vi "PathFollowingFinal.vi"(0 "GPS_Lat":dbl format="%#_13g", 5 "GPS_Long":dbl format="%#_13g", 7 "Path":dbl[][](array[numeric]), 9 "Heading angle":dbl, 11 "Save heading":bool=TRUE) -> (4 "Path rest":dbl[][](array[numeric]), 6 "Delta Heading Angle":dbl, 8 "Goal reached":bool, 10 "Beta":dbl format="%#_13g")   [LabVIEW 2016]
uses:
  <vilib>/express/express arith-compare/Formula/XNode/ExpressFormulaBlockNode.xnode
panel:
  out "Angle":dbl
  out "Distance":dbl format="%#.14g"
  out "Next Point":dbl[](array[numeric])
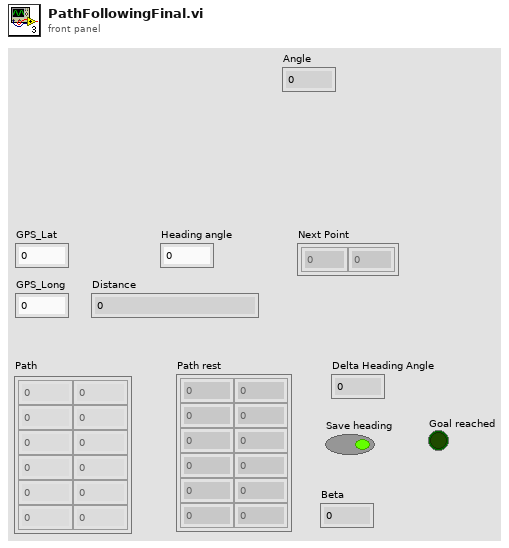
[diagram p1: front panel]
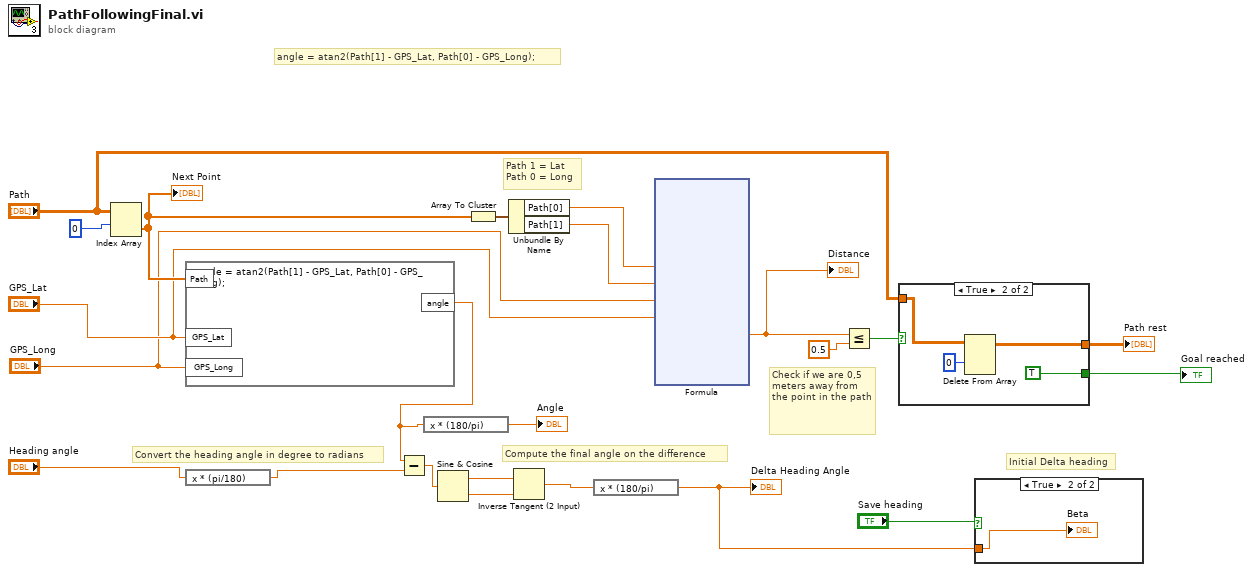
[diagram p0: block diagram]
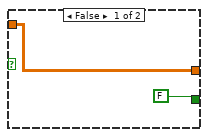
[diagram p3: hidden frame]
diagram:
  # "Initial Delta heading"
  # "angle = atan2(Path[1] - GPS_Lat, Path[0] - GPS_Long);"
  # "Convert the heading angle in degree to radians"
  # "Compute the final angle on the difference"
  # "Check if we are 0,5 meters away from the point in the path"
  # "Path 1 = Lat\nPath 0 = Long"
  n1 = Index Array(array="Path", index (row)=0) -> (element=w13:dbl[])  [unwired: 1 in]
  "Next Point" <- w13
  n2 = formula code="angle = atan2(Path[1] - GPS_Lat, Path[0] - GPS_Long);"("Path"=w13, "GPS_Long"="GPS_Long", "GPS_Lat"="GPS_Lat") -> ("angle"=w5:dbl)
  n3 = expression code="x * (pi/180)"("Heading angle") -> (w14:dbl)
  n4 = Subtract(x=w5, y=w14) -> (x-y=w16:dbl)
  n5 = expression code="x * (180/pi)"(w5) -> (→"Angle":dbl)
  n6 = Sine & Cosine(0:w16) -> (1:w19:dbl, 2:w18:dbl)
  n7 = Array To Cluster(array=w13) -> (cluster=w22:cluster{"Path[0]":dbl, "Path[1]":dbl})
  n8 = Unbundle By Name(w22) -> ("Path[0]"=w12:dbl, "Path[1]"=w11:dbl)
  n9 = Inverse Tangent (2 Input)(1:w18, 2:w19) -> (0:w17:dbl)
  n10 = expression code="x * (180/pi)"(w17) -> (w1:dbl)
  "Delta Heading Angle" <- w1
  n11 = xnode "Formula"("Path_LONG"=w12, "Path_LAT"=w11, "GPS_LONG"="GPS_Long", "GPS_LAT"="GPS_Lat") -> ("Result"=w8:dbl)  [unwired: 1 in, 1 out]
  "Distance" <- w8
  n12 = Less Or Equal?(x=w8, y=0.5) -> (x <= y?=w20:bool)
  n13 = case shown="True" w20 {
    tunnel: [w25 w28] -> w6
    tunnel: "Path" -> [w25 w27]
    tunnel: [FALSE TRUE] -> w3
    frame False {
    }
    frame True {
      n14 = Delete From Array(array=w27, index (row)=0) -> (array with subset deleted=w28:dbl[][])  [unwired: 2 in, 1 out]
    }
  }
  "Path rest" <- w6
  "Goal reached" <- w3
  n15 = case shown="True" "Save heading" {
    tunnel: w1 -> [_ w30]
    frame False {
    }
    frame True {
      "Beta" <- w30
    }
  }
